vi "ScaledWaveform-RemoveScaleParameterChannel.vi"(8 "Error in":errorcluster, 11 "Custom Device ref":T1 format="%.0x") -> (0 "Error out":errorcluster, 3 "Custom Device ref out":T1 format="%.0x")   [LabVIEW 2015, in "Waveform-Processing-Custom-Device Shared.lvlib" / "Scaled Waveform.lvlib"]
uses:
  Scaled Waveform.lvlib
  <vilib>/NI Veristand/Custom Device API/Custom Device Item Ref.ctl
  Constants.vi
  <vilib>/NI Veristand/Custom Device API/Get Item Property (Dependent Node Pointer).vi
  System Explorer/Waveform-Processing-Custom-Device System Explorer.lvlib
  <vilib>/NI VeriStand/Custom Device API/Custom Device API.lvlib
  Waveform-Processing-Custom-Device Shared.lvlib
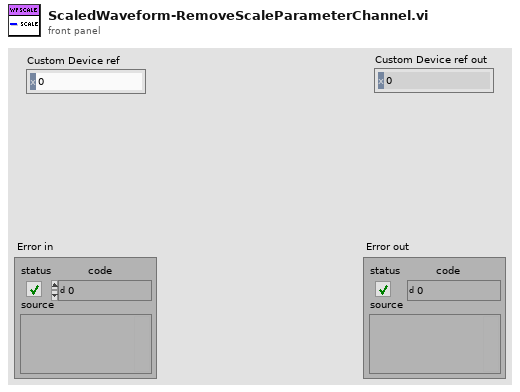
[diagram p1: front panel]
types:
  T1 = typedef "Custom Device API.lvlib/Custom Device Item Ref.ctl" = u64
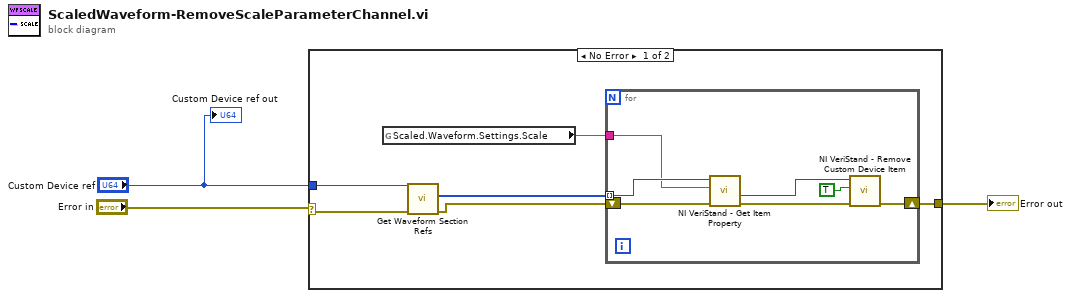
[diagram p0: block diagram]
diagram:
  n1 = case shown="No Error" "Error in" {
    selector: "Error in" -> [w9 w17]
    tunnel: "Custom Device ref" -> [w8 _]
    tunnel: [w5 w17] -> w2
    frame No Error {
      n2 = global read "Constants.vi" "Scaled.Waveform.Settings.Scale"() -> (w4:string)
      n3 = call "Get Waveform Section Refs.vi"("Error in"=w9, "Device Ref in"=w8) -> ("Error out"=w7:errorcluster, "Result Section Refs"=w6:T1[])  [unwired: 7 in, 1 out]
      n4 = for {
        tunnel: w6 -> [w13] mode=indexing
        shift-right: [w10] -> w5
        shift-left: w7 -> [w11]
        tunnel: w4 -> [w12]
        n5 = call-poly <vilib>:"NI VeriStand - Get Item Property.vi"("error in (no error)"=w11, "Property Name"=w12, "Item Ref in"=w13) -> ("error out"=w14:errorcluster, "Dependent Node Ref"=w15:T1)  [unwired: 5 in, 2 out]
        n6 = call <vilib>:"NI VeriStand - Remove Custom Device Item.vi"("error in (no error)"=w14, "Force Delete (F)"=TRUE, "Item Ref in"=w15) -> ("error out"=w10:errorcluster)  [unwired: 7 in, 1 out]
      }
    }
    frame Error {
    }
  }
  "Error out" <- w2
  "Custom Device ref out" <- "Custom Device ref"
